vi "GLIMPSE Sequence Save.vi"(5 "Go? (F)":bool, 6 "Header file data":T1 {"Pixel depth" items=["8 bits", "16 bits", "Float", "Complex", "RGB", "HSL"]; "time of 1st frame, \nsec since 1/1/04" format="%.2f"}, 8 "Acquisition refnum array":refnum<file>[](array[refnum]), 9 "Black/White Levels":cluster{ext, ext}(slide)={1.0, 65535.0} scale=1.0..65535.0) -> ()   [LabVIEW 2011]
doc: "Saves a sequence either as a single movied file (SEQ, Stacked TIFF, or AVI) or as a directory full of individual frame images (Multiple TIFF). If more than one AOI is specified, each is saved in a separate, sequentially numbered file or directory. For stacked TIFF or AVI formats, also saves a separate .mat file with time information etc. See Save sequence file into movie.vi for information on the file format."
uses:
  Header file data.ctl
  Seq file v 1/Offset table.ctl
  Seq file v 1/Offset.ctl
  Seq file v 1/file number.ctl
  GLIMPSE Globals.vi
  AOI/AOI List Globals.vi
panel:
  in  "AVI AOI Overlay\n(\"Entire Frames\" only)":bool
  in  "AVI Frames Per Second":u32=30
  out "Keep acquisition files open at end":bool=TRUE
  in  "Change File":bool
  out "Current movie directory":path=path "d:/1.glimpse"
  in  "AOI Options":i32(listbox)=1
  in  "stop":bool
  in  "Description Info (SEQ and stacked TIFF formats)":string
  in  "To":u32
  in  "From":u32
  in  "Frame Range Options":i32(listbox)
  in  "File Format Options":i32(listbox)
  # "Make any changes required, then press"
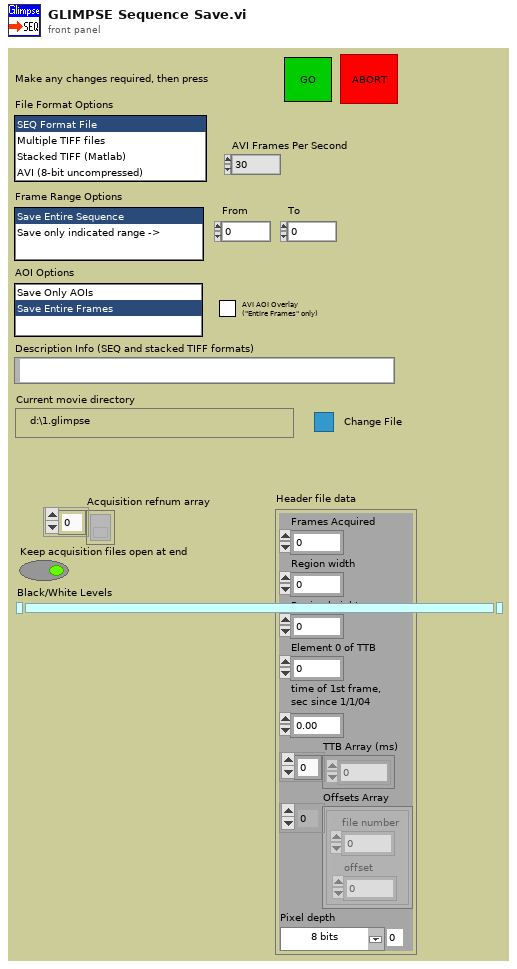
[diagram p1: front panel]
types:
  T1 = typedef "Header file data.ctl" = cluster{"Frames Acquired":u32, "Region width":i32, "Region height":i32, "Element 0 of TTB":u32, "time of 1st frame, \nsec since 1/1/04":dbl, "TTB Array (ms)":u32[], "Offsets Array":T2, "Pixel depth":u32}
  T2 = typedef "Offset table.ctl" = cluster{"offset":T3, "file number":T4}[]
  T3 = typedef "Offset.ctl" = i32
  T4 = typedef "file number.ctl" = u8
  T5 = enum16{"Frames", "Fields, Odd 1st", "Fields, Even 1st", "Fields, Averaged"}
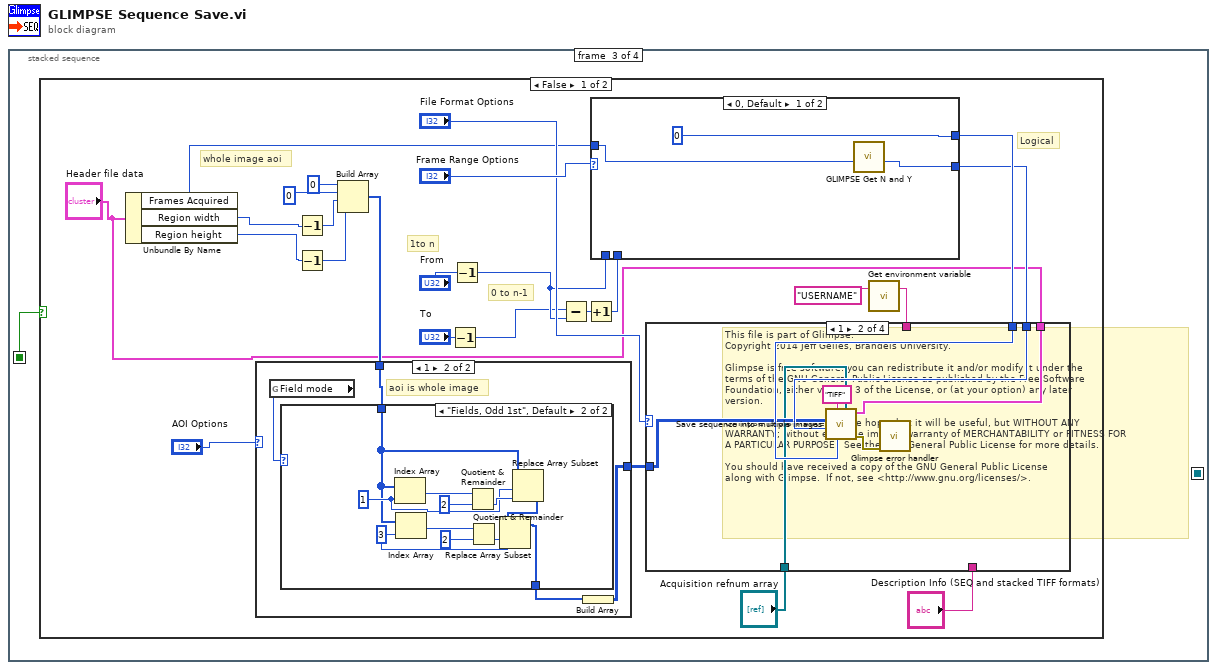
[diagram p0: block diagram]
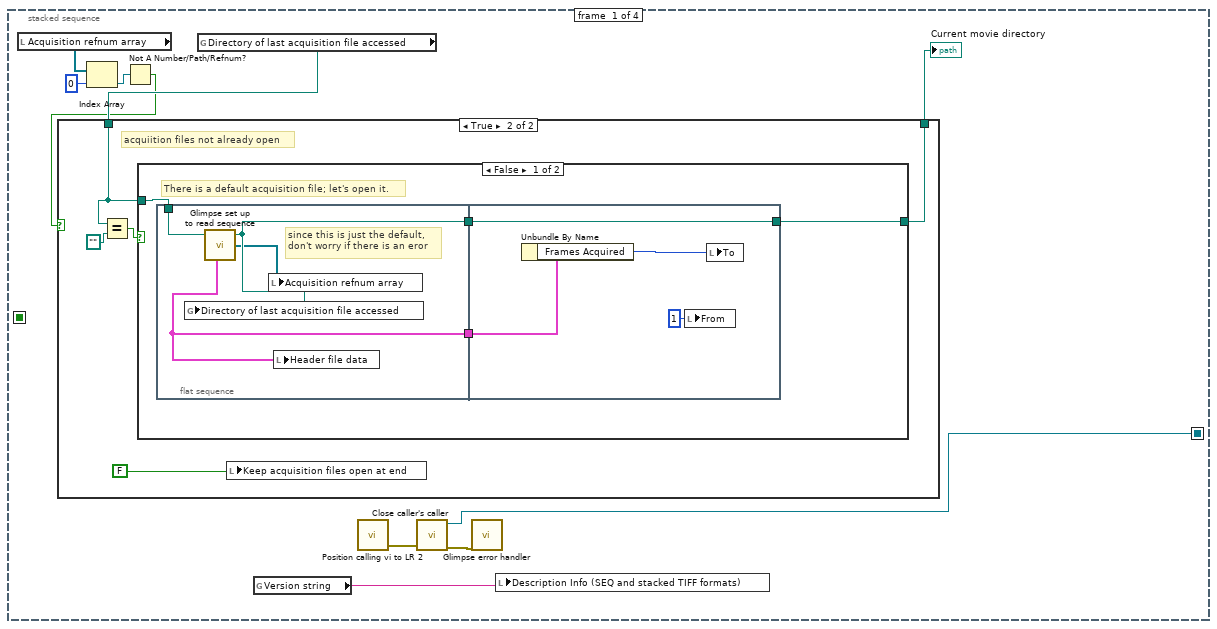
[diagram p2: hidden frame]
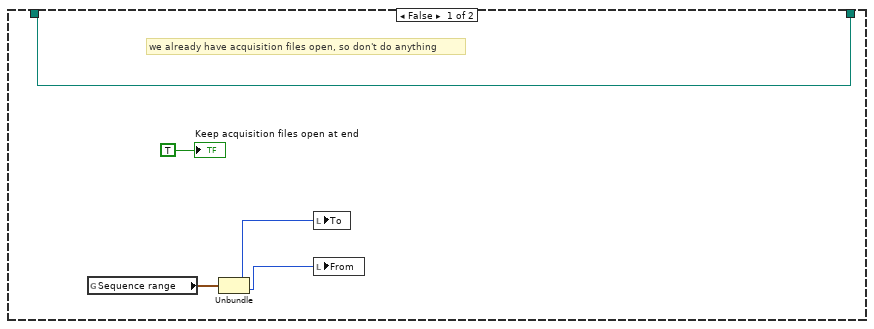
[diagram p3: hidden frame]
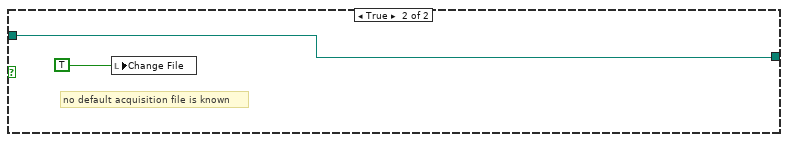
[diagram p4: hidden frame]
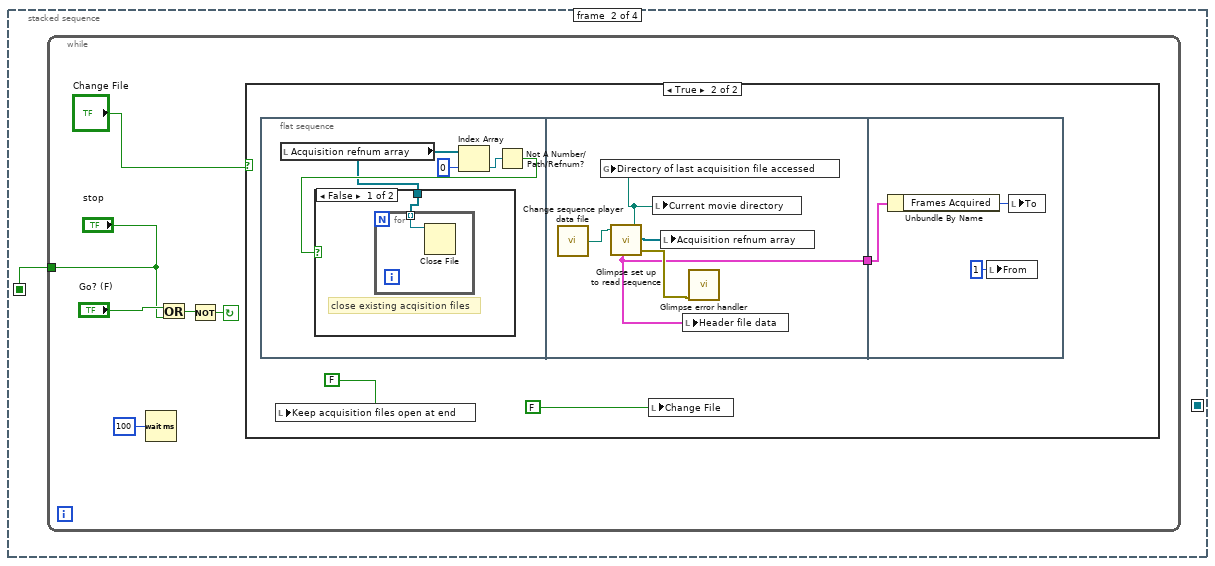
[diagram p5: hidden frame]
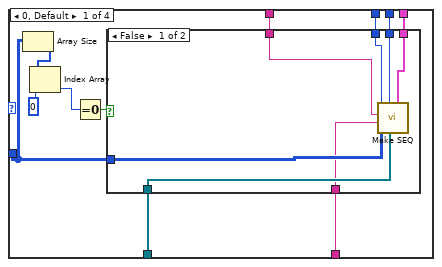
[diagram p8: hidden frame]
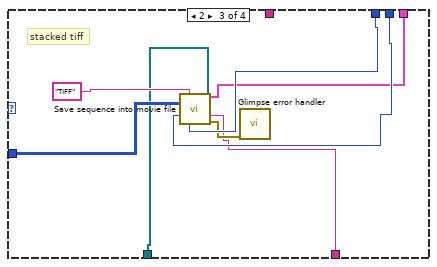
[diagram p10: hidden frame]
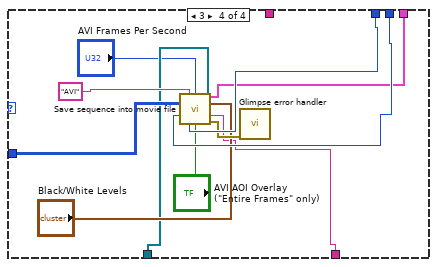
[diagram p11: hidden frame]
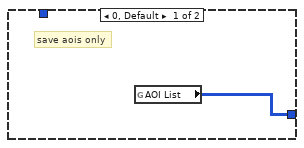
[diagram p12: hidden frame]
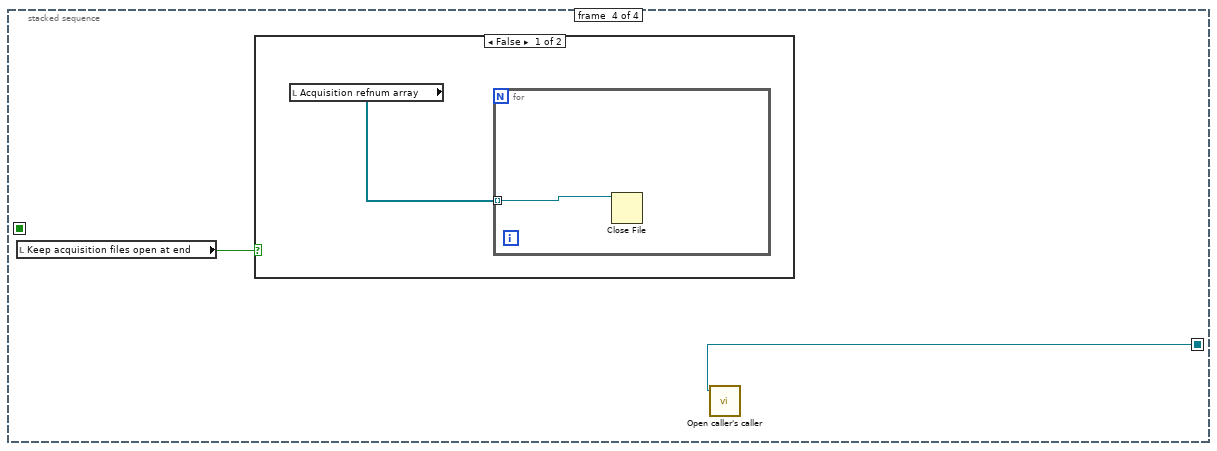
[diagram p16: hidden frame]
diagram:
  # "This file is part of Glimpse. \nCopyright 2014 Jeff Gelles, Brandeis University.    \n\nGlimpse is free software: you can redistribute it and/or modify it under the \nterms of the GNU General Public License as published by the Free Software \nFoundation, either version 3 of the License, or (at your option) any later \nversion.\n\nGlimpse is distributed in the hope that it will be useful, but WITHOUT ANY \nWARRANTY; without even the implied warranty of MERCHANTABILITY or FITNESS FOR \nA PARTICULAR PURPOSE.  See the GNU General Public License for more details.\n\nYou should have received a copy of the GNU General Public License\nalong with Glimpse.  If not, see <http://www.gnu.org/licenses/>."
  n1 = stacked-sequence {
    seq-local: [_ w35 _ _] -> [_ _ w59 _]
    seq-local: [w1 _ _ _] -> [_ _ _ w151]
    frame #0 {
      n2 = local read "Acquisition refnum array"() -> (w8:refnum<file>[])
      n3 = Index Array(array=w8, index=0) -> (element=w6:refnum<file>)
      n4 = Not A Number/Path/Refnum?(number/path/refnum=w6) -> (NaN/Path/Refnum?=w5:bool)
      n5 = global read "GLIMPSE Globals.vi" "Directory of last acquisition file accessed"() -> (w10:path)
      n6 = case shown="True" w5 {
        tunnel: w10 -> [w15 w18]
        tunnel: [w15 w17] -> w9
        frame False {
          # "we already have acquisition files open, so don't do anything"
          n7 = global read "GLIMPSE Globals.vi" "Sequence range"() -> (w13:cluster{i16, i16})
          n8 = Unbundle(w13) -> (w12:i16, w11:i16)
          n9 = local write "To"(w12) -> ()
          n10 = local write "From"(w11) -> ()
          "Keep acquisition files open at end" <- TRUE
        }
        frame True {
          # "acquiition files not already open"
          n11 = Equal?(x=w18, y=path "") -> (x = y?=w19:bool)
          n12 = case shown="False" w19 {
            tunnel: w18 -> [w24 w33]
            tunnel: [w23 w33] -> w17
            frame False {
              # "There is a default acquisition file; let's open it."
              n13 = flat-sequence {
                tunnel: w24 -> [w28]
                tunnel: [w27] -> w22
                tunnel: [w25] -> w21
                tunnel: [w31] -> w23
                tunnel: w22 -> [w31]
                tunnel: w21 -> [w30]
                frame #0 {
                  # "since this is just the default,\ndon't worry if there is an eror"
                  n14 = call "Glimpse set up to read sequence.vi"("acquisition directory path"=w28) -> ("Header file data out"=w25:T1, "acquisition directory path out"=w27:path, "Acquisition refnum array"=w26:refnum<file>[])  [unwired: 1 in, 3 out]
                  n15 = global write "GLIMPSE Globals.vi" "Directory of last acquisition file accessed"(w27) -> ()
                  n16 = local write "Acquisition refnum array"(w26) -> ()
                  n17 = local write "Header file data"(w25) -> ()
                }
                frame #1 {
                  n18 = Unbundle By Name(w30) -> ("Frames Acquired"=w29:u32)
                  n19 = local write "From"(u16 1 ("From")) -> ()
                  n20 = local write "To"(w29) -> ()
                }
              }
            }
            frame True {
              # "no default acquisition file is known"
              n21 = local write "Change File"(TRUE) -> ()
            }
          }
          n22 = local write "Keep acquisition files open at end"(FALSE) -> ()
        }
      }
      "Current movie directory" <- w9
      n23 = global read "GLIMPSE Globals.vi" "Version string"() -> (w4:string)
      n24 = call "Position calling vi to LR 2.vi"() -> ("error out"=w3:errorcluster)  [unwired: 2 in, 3 out]
      n25 = call "Close caller's caller.vi"("error in (no error)"=w3) -> ("error out"=w2:errorcluster, "vi reference"=w1:refnum<vi>)  [unwired: 6 out]
      n26 = call "Glimpse error handler.vi"("error in"=w2) -> ()  [unwired: 1 in, 6 out]
      n27 = local write "Description Info (SEQ and stacked TIFF formats)"(w4) -> ()
    }
    frame #1 {
      n28 = while {
        tunnel: ["stop"] -> w35
        stop <- w40 continue-if-true
        n29 = Wait (ms)(milliseconds to wait=u32 100) -> ()  [unwired: 1 out]
        n30 = Or(x="Go? (F)", y="stop") -> (x .or. y?=w38:bool)
        n31 = Not(x=w38) -> (.not. x?=w40:bool)
        n32 = case shown="True" "Change File" {
          frame False {
          }
          frame True {
            n33 = flat-sequence {
              tunnel: [w51] -> w42
              tunnel: w42 -> [w57]
              frame #0 {
                n34 = local read "Acquisition refnum array"() -> (w45:refnum<file>[])
                n35 = Index Array(array=w45, index=0) -> (element=w47:refnum<file>)
                n36 = Not A Number/Path/Refnum?(number/path/refnum=w47) -> (NaN/Path/Refnum?=w46:bool)
                n37 = case shown="False" w46 {
                  tunnel: w45 -> [w49 _]
                  frame False {
                    # "close existing acqisition files"
                    n38 = for {
                      tunnel: w49 -> [w50] mode=indexing
                      n39 = Close File(refnum=w50) -> ()  [unwired: 1 in, 2 out]
                    }
                  }
                  frame True {
                  }
                }
              }
              frame #1 {
                n40 = call "Change sequence player data file.vi"() -> ("File path out"=w55:path)  [unwired: 1 in, 4 out]
                n41 = call "Glimpse set up to read sequence.vi"("acquisition directory path"=w55) -> ("Header file data out"=w51:T1, "acquisition directory path out"=w54:path, "Acquisition refnum array"=w53:refnum<file>[], "error out"=w52:errorcluster)  [unwired: 1 in, 2 out]
                n42 = global write "GLIMPSE Globals.vi" "Directory of last acquisition file accessed"(w54) -> ()
                n43 = local write "Current movie directory"(w54) -> ()
                n44 = local write "Acquisition refnum array"(w53) -> ()
                n45 = local write "Header file data"(w51) -> ()
                n46 = call "Glimpse error handler.vi"("error in"=w52) -> ()  [unwired: 1 in, 6 out]
              }
              frame #2 {
                n47 = Unbundle By Name(w57) -> ("Frames Acquired"=w56:u32)
                n48 = local write "From"(u16 1 ("From")) -> ()
                n49 = local write "To"(w56) -> ()
              }
            }
            n50 = local write "Keep acquisition files open at end"(FALSE) -> ()
            n51 = local write "Change File"(FALSE) -> ()
          }
        }
      }
    }
    frame #2 {
      n52 = case shown="False" w59 {
        frame False {
          # "0 to n-1"
          # "1to n"
          # "whole image aoi"
          # "Logical"
          n53 = Unbundle By Name("Header file data") -> ("Frames Acquired"=w65:u32, "Region width"=w67:i32, "Region height"=w66:i32)
          n54 = Decrement(x=w67) -> (x-1=w71:i32)
          n55 = Decrement(x=w66) -> (x-1=w69:i32)
          n56 = Build Array(u16 0 ("element"), u16 0 ("element"), w71, w69) -> (w68:i32[])
          n57 = case shown="1" "AOI Options" {
            tunnel: [w129 w133] -> w79
            tunnel: w68 -> [_ w130]
            frame 0, Default {
              # "save aois only"
              n58 = global read "AOI List Globals.vi" "AOI List"() -> (w129:u16[][])
            }
            frame 1 {
              # "aoi is whole image"
              n59 = global read "GLIMPSE Globals.vi" "Field mode"() -> (w132:T5)
              n60 = case shown="\"Fields, Odd 1st\", Default" w132 {
                tunnel: [w134 w138] -> w131
                tunnel: w130 -> [w134 w135]
                frame "Frames" {
                }
                frame "Fields, Odd 1st", Default {
                  w143 = 3 ("Index")
                  w139 = 1 ("Index")
                  n61 = Index Array(array=w135, index=w139) -> (element=w137:i32)
                  n62 = Index Array(array=w135, index=w143) -> (element=w136:i32)
                  n63 = Quotient & Remainder(x=w137, y=i8 2) -> (floor(x/y)=w144:i32)  [unwired: 1 out]
                  n64 = Quotient & Remainder(x=w136, y=i8 2) -> (floor(x/y)=w140:i32)  [unwired: 1 out]
                  n65 = Replace Array Subset(array=w135, new element=w144, index=w139) -> (w141:i32[])
                  n66 = Replace Array Subset(array=w141, new element=w140, index=w143) -> (w138:i32[])
                }
              }
              n67 = Build Array(w131) -> (w133:i32[][])
            }
          }
          n68 = Decrement(x="To") -> (x-1=w75:u32)
          n69 = Decrement(x="From") -> (x-1=w76:u32)
          n70 = Subtract(x=w75, y=w76) -> (x-y=w83:u32)
          n71 = Increment(x=w83) -> (x+1=w82:u32)
          n72 = case shown="0, Default" "Frame Range Options" {
            tunnel: w76 -> [_ w150]
            tunnel: w82 -> [_ w149]
            tunnel: [u32 0 w150] -> w74
            tunnel: [w147 w149] -> w73
            tunnel: w65 -> [w146 _]
            frame 0, Default {
              n73 = call "GLIMPSE Get N and Y.vi"("# of Frames In (Phys)"=w146) -> ("# of Frames Out (Log)"=w147:u32)  [unwired: 2 in, 4 out]
            }
            frame 1 {
            }
          }
          n74 = call "Get environment variable.vi"("Variable name"="USERNAME") -> ("Value"=w60:string)  [unwired: 2 out]
          n75 = case shown="1" "File Format Options" {
            tunnel: w79 -> [w95 w105 w117 w128]
            tunnel: w73 -> [w90 w107 w113 w124]
            tunnel: w74 -> [w89 w108 w116 w127]
            tunnel: "Header file data" -> [w88 w104 w112 w123]
            tunnel: "Acquisition refnum array" -> [w87 w103 w111 w121]
            tunnel: "Description Info (SEQ and stacked TIFF formats)" -> [w86 _ w110 w120]
            tunnel: w60 -> [w85 _ _ _]
            frame 0, Default {
              n76 = Array Size(array=w95) -> (size(s)=w94:i32[])
              n77 = Index Array(array=w94, index=0) -> (element=w92:i32)
              n78 = Equal To 0?(x=w92) -> (x = 0?=w91:bool)
              n79 = case shown="False" w91 {
                tunnel: w95 -> [w102 _]
                tunnel: w90 -> [w100 _]
                tunnel: w89 -> [w101 _]
                tunnel: w88 -> [w99 _]
                tunnel: w87 -> [w98 _]
                tunnel: w86 -> [w97 _]
                tunnel: w85 -> [w96 _]
                frame False {
                  n80 = call "Make SEQ.vi"("Header file data"=w99, "Acqisition files refnums"=w98, "Number of images"=w100, "AOI List"=w102, "Description"=w97, "User Info"=w96, "First image number (start 0)"=w101) -> ()  [unwired: 1 in, 3 out]
                }
                frame True {
                }
              }
            }
            frame 1 {
              n81 = call "Save sequence into multiple images.vi"("Header file data"=w104, "Acqisition files refnums"=w103, "starting frame number to save"=w108, "File Format"="TIFF" ("File Type"), "Number of frames to save"=w107, "AOI List"=w105) -> ("error out"=w106:errorcluster)  [unwired: 2 in, 2 out]
              n82 = call "Glimpse error handler.vi"("error in"=w106) -> ()  [unwired: 1 in, 6 out]
            }
            frame 2 {
              # "stacked tiff"
              n83 = call "Save sequence into movie file.vi"("File Format"="TIFF" ("File Type"), "Header file data"=w112, "AOI List"=w117, "Acqisition files refnums"=w111, "Number of frames to save"=w113, "Description Info (SEQ and stacked TIFF formats)"=w110, "starting frame number to save"=w116) -> ("error out"=w115:errorcluster)  [unwired: 5 in, 3 out]
              n84 = call "Glimpse error handler.vi"("error in"=w115) -> ()  [unwired: 1 in, 6 out]
            }
            frame 3 {
              n85 = call "Save sequence into movie file.vi"("File Format"="AVI" ("File Type"), "AVI Frames Per Second"="AVI Frames Per Second", "Header file data"=w123, "AOI List"=w128, "Black/White Levels"="Black/White Levels", "Acqisition files refnums"=w121, "Number of frames to save"=w124, "Description Info (SEQ and stacked TIFF formats)"=w120, "starting frame number to save"=w127, "AOI Overlay?"="AVI AOI Overlay\n(\"Entire Frames\" only)") -> ("error out"=w126:errorcluster)  [unwired: 2 in, 3 out]
              n86 = call "Glimpse error handler.vi"("error in"=w126) -> ()  [unwired: 1 in, 6 out]
            }
          }
        }
        frame True {
        }
      }
    }
    frame #3 {
      n87 = local read "Keep acquisition files open at end"() -> (w152:bool)
      n88 = case shown="False" w152 {
        frame False {
          n89 = local read "Acquisition refnum array"() -> (w153:refnum<file>[])
          n90 = for {
            tunnel: w153 -> [w154] mode=indexing
            n91 = Close File(refnum=w154) -> ()  [unwired: 1 in, 2 out]
          }
        }
        frame True {
        }
      }
      n92 = call "Open caller's caller.vi"("vi reference"=w151) -> ()  [unwired: 1 in, 7 out]
    }
  }
